vi "Celcius 2 Fahrenheit.vi"() -> ()   [LabVIEW 2019]
panel:
  out "F":dbl
  in  "C":dbl
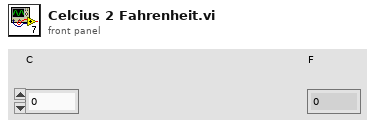
[diagram p1: front panel]
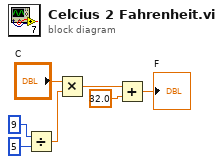
[diagram p0: block diagram]
diagram:
  n1 = Divide(x=9, y=5) -> (x/y=w1:dbl)
  n2 = Multiply(x="C", y=w1) -> (x*y=w5:dbl)
  n3 = Add(x=w5, y=32.0) -> (x+y=→"F":dbl)
